vi "Session Async.vi"(10 "ExecAnchor":refnum<class "ExecAnchor.lvclass">, 11 "Promise":refnum<class "Promise.lvclass">) -> ()   [LabVIEW 2020, in "User Prefs.lvlib" / "PrefsDB.lvclass"]
uses:
  PrefsDB.lvclass
  lv-exec-anchor/ExecAnchor/ExecAnchor.lvclass
  PrefsDB.lvclass/PrefsDB.ctl
  C:/dev/lv20CE/relink/lv-promises/Promises/Value/Value.lvclass
  Pref Group/Pref Group.lvclass
  lv-promises/Promises/Promise/Promise.lvclass
  Obtain Group Data.ctl
  lv-cdm/CDM-Config/Config Manager/Config Manager.lvclass
  Write Pref Data.ctl
  User Prefs.lvlib
  lv-cdm/CDM-Config/Config Element/Config Element.lvclass
  C:/dev/lv20CE/relink/lv-userprefs/User Prefs/PrefsDB/PrefsDB.lvclass
  lv-promises/Promises/No Parameter/No Parameter.lvclass
  C:/dev/lv20CE/relink/lv-userprefs/User Prefs/Pref Group/Pref Group.lvclass
  C:/dev/lv20CE/relink/lv-promises/Promises/No Parameter/No Parameter.lvclass
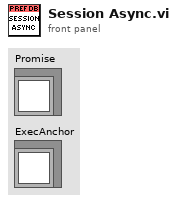
[diagram p1: front panel]
types:
  T1 = cluster{"ExecAnchor":refnum<event-registration>, "PrefDB":refnum<event-registration>}
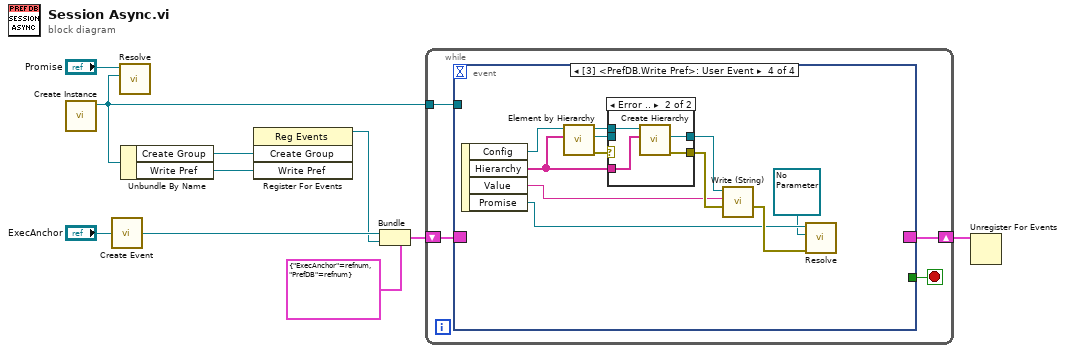
[diagram p0: block diagram]
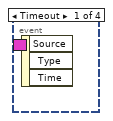
[diagram p2: hidden frame]
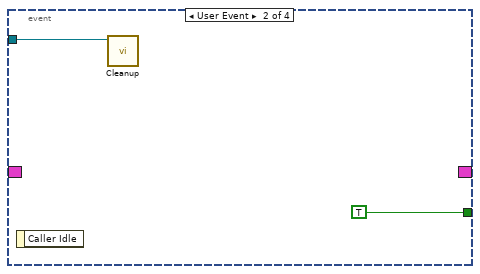
[diagram p3: hidden frame]
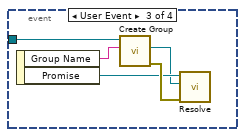
[diagram p4: hidden frame]
diagram:
  n1 = call "Create Instance.vi"() -> ("PrefsDB out"=w6:refnum<class "PrefsDB.lvclass">)  [unwired: 10 in, 1 out]
  n2 = call "Create Event.vi"("ExecAnchor in"="ExecAnchor") -> ("Event Reg"=w8:refnum<event-registration>)  [unwired: 3 in, 1 out]
  n3 = call "Resolve.vi"("Result"=w6, "Promise in"="Promise") -> ()  [unwired: 8 in, 2 out]
  n4 = Unbundle By Name(w6) -> ("Create Group"=w5:refnum<user-event>, "Write Pref"=w2:refnum<user-event>)
  n5 = register-events(w5, w2) -> (reference out=w4:refnum<event-registration>)  [unwired: 2 in, 1 out]
  n6 = Bundle(cluster=T1 {"ExecAnchor"=refnum, "PrefDB"=refnum}, "ExecAnchor"=w8, "PrefDB"=w4) -> (w3:T1)
  n7 = while {
    shift-right: [w13] -> w7
    shift-left: w3 -> [w14]
    tunnel: w6 -> [w12]
    stop <- w11 stop-if-true
    n8 = event shown="[3] <PrefDB.Write Pref>: User Event" {
      selector: w14 -> [_ _ _ _]
      dyn-events: [_ _ _ _] -> w13
      timeout: _ -> [_ _ _ _]
      tunnel: w12 -> [_ w16 w19 _]
      tunnel: [_ TRUE _ _] -> w11
      event Timeout {
        n9 = event-data() -> ()  [unwired: 1 in, 3 out]
      }
      event User Event {
        n10 = event-data() -> ()  [unwired: 1 in, 1 out]
        n11 = call "Cleanup.vi"("PrefsDB in"=w16) -> ()  [unwired: 10 in, 1 out]
      }
      event User Event {
        n12 = event-data() -> ("Group Name"=w18:string, "Promise"=w20:refnum<class "Promise.lvclass">)  [unwired: 1 in]
        n13 = call "Create Group.vi"("Group"=w18, "PrefsDB in"=w19) -> ("error out"=w21:errorcluster, "Pref Group"=w17:refnum<class "Pref Group.lvclass">)  [unwired: 7 in, 1 out]
        n14 = call "Resolve.vi"("error in (no error)"=w21, "Result"=w17, "Promise in"=w20) -> ()  [unwired: 7 in, 2 out]
      }
      event User Event {
        n15 = event-data() -> ("Config"=w26:refnum<class "Config Manager.lvclass">, "Hierarchy"=w25:string[], "Value"=w24:string, "Promise"=w23:refnum<class "Promise.lvclass">)  [unwired: 1 in]
        n16 = call "Element by Hierarchy.vi"("Hierarchy"=w25, "Config Manager in"=w26) -> ("error out"=w31:errorcluster, "Config Element"=w30:refnum<class "Config Element.lvclass">, "Config Manager out"=w29:refnum<class "Config Manager.lvclass">)  [unwired: 7 in]
        n17 = case shown="Error .." w31 {
          tunnel: w30 -> [w33 _]
          tunnel: [w33 w35] -> w28
          tunnel: w29 -> [_ w37]
          tunnel: w25 -> [_ w36]
          tunnel: [_ w34] -> w27
          frame No Error {
          }
          frame Error {
            n18 = call "Create Hierarchy.vi"("Hierarchy"=w36, "Config Manager in"=w37) -> ("error out"=w34:errorcluster, "Leaf Element"=w35:refnum<class "Config Element.lvclass">)  [unwired: 7 in, 1 out]
          }
        }
        n19 = call "Write (String).vi"("error in (no error)"=w27, "String Value"=w24, "Config Element in"=w28) -> ("error out"=w32:errorcluster)  [unwired: 7 in, 1 out]
        n20 = call "Resolve.vi"("error in (no error)"=w32, "Result"=refnum<class "No Parameter.lvclass"> refnum ("Futures:No Parameter.lvclass"), "Promise in"=w23) -> ()  [unwired: 7 in, 2 out]
      }
    }
  }
  n21 = Unregister For Events(event registration refnum=w7) -> ()  [unwired: 1 in, 1 out]
